vi "FlatSequenceInnerTunnel.vi"(8 "error in":errorcluster, 11 "reference":refnum<vi>) -> (0 "error out":errorcluster, 3 "Tunnel out":refnum<class "FlatSequenceInnerTunnel.lvclass">)   [LabVIEW 2014, in "Raspberry Pi Compatible Compiler for LabVIEW.lvlib" / "FlatSequenceInnerTunnel.lvclass"]
uses:
  FlatSequenceInnerTunnel.lvclass
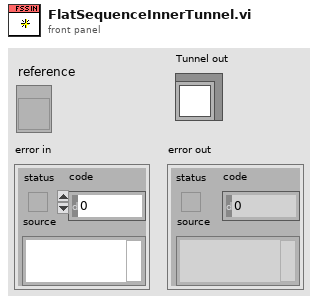
[diagram p1: front panel]
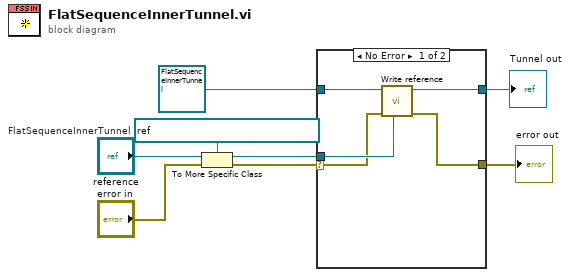
[diagram p0: block diagram]
diagram:
  w7 = refnum<vi> refnum  # FlatSequenceInnerTunnel
  n1 = To More Specific Class(target class=w7, reference="reference", error in="error in") -> (specific class reference=w1:refnum<vi>, error out=w5:errorcluster)
  n2 = case shown="No Error" w5 {
    selector: w5 -> [w10 w14]
    tunnel: refnum<class "FlatSequenceInnerTunnel.lvclass"> refnum ("Tunnel in") -> [w13 w15]
    tunnel: [w12 w15] -> w3
    tunnel: [w9 w14] -> w2
    tunnel: w1 -> [w11 _]
    frame No Error {
      n3 = call-dynamic "Write reference.vi"("reference"=w11, "error in"=w10, "GObject in"=w13) -> ("error out"=w9:errorcluster, "GObject out"=w12:refnum<class "FlatSequenceInnerTunnel.lvclass">)  [unwired: 5 in]
    }
    frame Error {
    }
  }
  "error out" <- w2
  "Tunnel out" <- w3
